vi "sub vi - Read Analog All v9.4.vi"() -> (0 "DATA0":dbl[](graph), 2 "Analog loop time":dbl, 3 "array GRAPH":dynamicdata[](array[waveform]), 4 "LAB01":T2, 5 "DATA1":dbl[](graph), 6 "LAB02":T3, 7 "DATA2":dbl[](graph), 8 "LAB03":T4, 10 "LAB04":T5, 13 "deg C":dbl, 14 "USB Error":bool[](array[boolean]), 15 "LAB05":T6)   [LabVIEW 2013]
uses:
  <vilib>/addons/Electrical Power/Basic/NI_EP_Basic.lvlib
  <vilib>/addons/Electrical Power/Basic/Measurement/Power (1 Channel).vi
  <vilib>/addons/Electrical Power/Basic/Measurement/RMS (N Channels).vi
  <vilib>/measure/NI_MAPro.lvlib
  <vilib>/measure/mascope.llb/Amplitude and Levels 1 chan.vi
  program files/Global display 3.vi
  <vilib>/addons/Electrical Power/Basic/Measurement/RMS (1 Channel).vi
panel:
  in  "Tab Control":T1(tab)
  out "LAB01-2 (PF)":dbl
  out "LAB01-1 (PF)":dbl
  out "LAB01-2 (V)":dbl
  out "LAB01-2 (A)":dbl
  out "LAB01-1 (V)":dbl
  out "LAB01-1 (A)":dbl
  out "LAB01-2 (GRAPH)":dynamicdata(graph)
  out "LAB01-1 (GRAPH)":dynamicdata(graph)
  out "LAB02-2 (PF)":dbl
  out "LAB02-1 (PF)":dbl
  out "LAB02-2 (V)":dbl
  out "LAB02-2 (A)":dbl
  out "LAB02-1 (V)":dbl
  out "LAB02-1 (A)":dbl
  out "LAB02-2 (GRAPH)":dynamicdata(graph)
  out "LAB02-1 (GRAPH)":dynamicdata(graph)
  out "LAB03-2 (PF)":dbl
  out "LAB03-1 (PF)":dbl
  out "LAB03-2 (V)":dbl
  out "LAB03-2 (A)":dbl
  out "LAB03-1 (V)":dbl
  out "LAB03-1 (A)":dbl
  out "LAB03-2 (GRAPH)":dynamicdata(graph)
  out "LAB03-1 (GRAPH)":dynamicdata(graph)
  out "LAB04-2 (PF)":dbl
  out "LAB04-1 (PF)":dbl
  out "LAB04-2 (V)":dbl
  out "LAB04-2 (A)":dbl
  out "LAB04-1 (V)":dbl
  out "LAB04-1 (A)":dbl
  out "LAB04-1 (GRAPH)":dynamicdata(graph)
  out "LAB04-2 (GRAPH)":dynamicdata(graph)
  out "LAB05-2 (PF)":dbl
  out "LAB05-1 (PF)":dbl
  out "LAB05-2 (V)":dbl
  out "LAB05-2 (A)":dbl
  out "LAB05-1 (V)":dbl
  out "LAB05-1 (A)":dbl
  out "LAB05-1 (GRAPH)":dynamicdata(graph)
  out "LAB05-2 (GRAPH)":dynamicdata(graph)
  out "A1 error":errorcluster
  out "array ERROR":errorcluster[](array[cluster])
  out "AI2-OFF":waveform(dbl)[](graph)
  out "AI2-ON":waveform(dbl)[](graph)
  out "AI1-OFF":waveform(dbl)[](graph)
  out "AI1-ON":waveform(dbl)[](graph)
  out "AI0-OFF":waveform(dbl)[](graph)
  out "AI0-ON":waveform(dbl)[](graph)
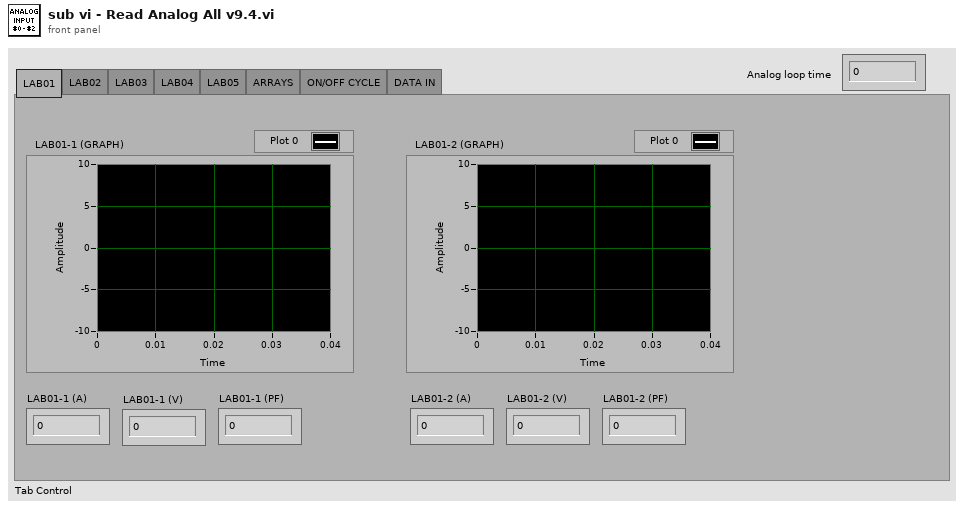
[diagram p1: front panel]
types:
  T1 = enum32{"LAB01", "LAB02", "LAB03", "LAB04", "LAB05", "ARRAYS", "ON/OFF CYCLE", "DATA IN"}
  T2 = cluster{"LAB01-1 (A)":dbl, "LAB01-1 (V)":dbl, "LAB01-1 (PF)":dbl, "LAB01-2 (A)":dbl, "LAB01-2 (V)":dbl, "LAB01-2 (PF)":dbl}
  T3 = cluster{"LAB02-1 (A)":dbl, "LAB02-1 (V)":dbl, "LAB02-1 (PF)":dbl, "LAB02-2 (A)":dbl, "LAB02-2 (V)":dbl, "LAB02-2 (PF)":dbl}
  T4 = cluster{"LAB03-1 (A)":dbl, "LAB03-1 (V)":dbl, "LAB03-1 (PF)":dbl, "LAB03-2 (A)":dbl, "LAB03-2 (V)":dbl, "LAB03-2 (PF)":dbl}
  T5 = cluster{"LAB04-1 (A)":dbl, "LAB04-1 (V)":dbl, "LAB04-1 (PF)":dbl, "LAB04-2 (A)":dbl, "LAB04-2 (V)":dbl, "LAB04-2 (PF)":dbl}
  T6 = cluster{"LAB05-1 (A)":dbl, "LAB05-1 (V)":dbl, "LAB05-1 (PF)":dbl, "LAB05-2 (A)":dbl, "LAB05-2 (V)":dbl, "LAB05-2 (PF)":dbl}
  T7 = typedef "NI_EP_Basic.lvlib/basic_Power Value.ctl" = cluster{"active power [W]":dbl, "apparent power [VA]":dbl, "reactive power [VAR]":dbl, "power factor":dbl}
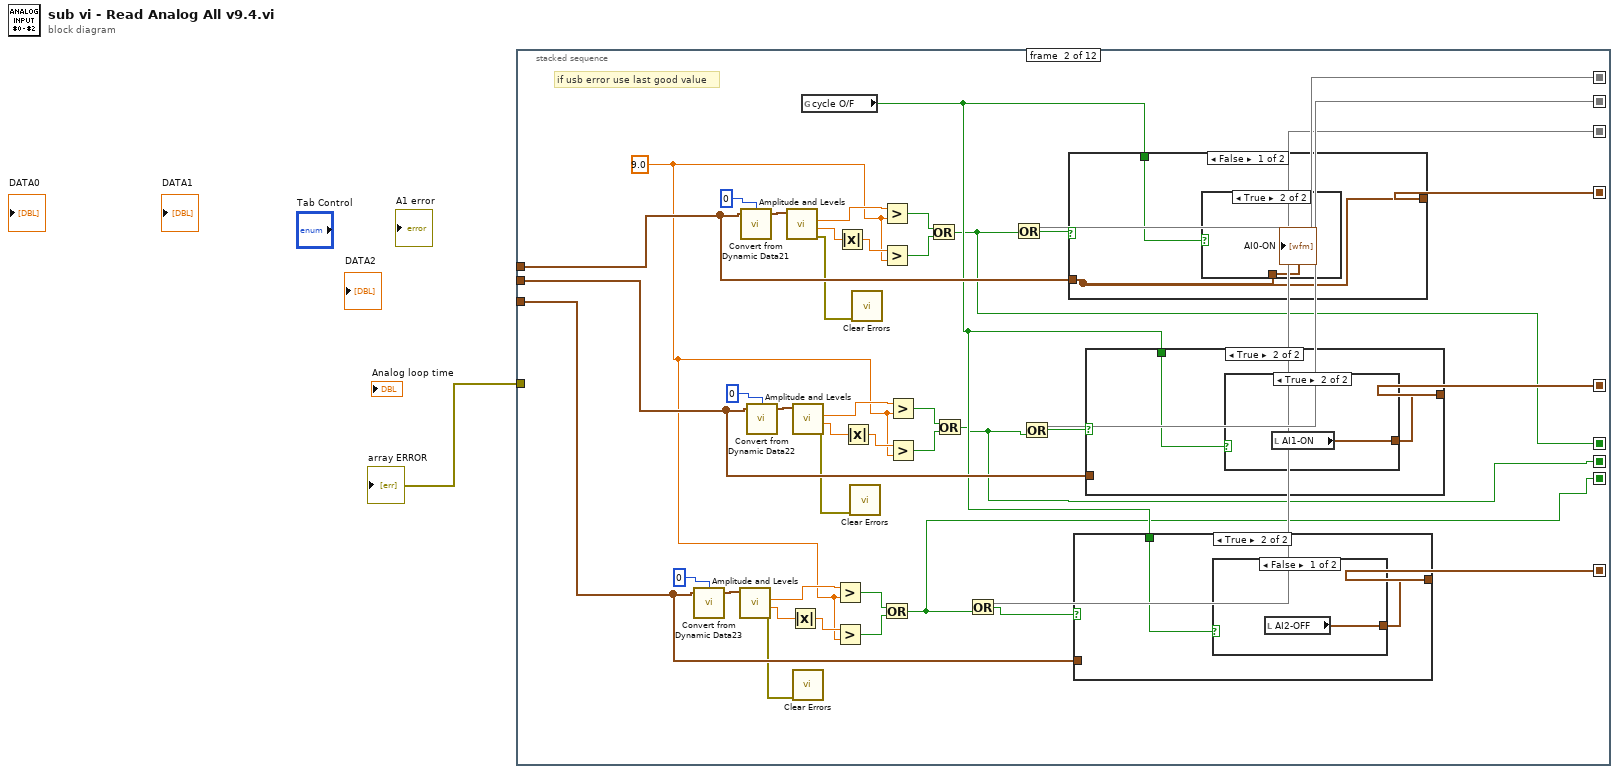
[diagram p0: block diagram]
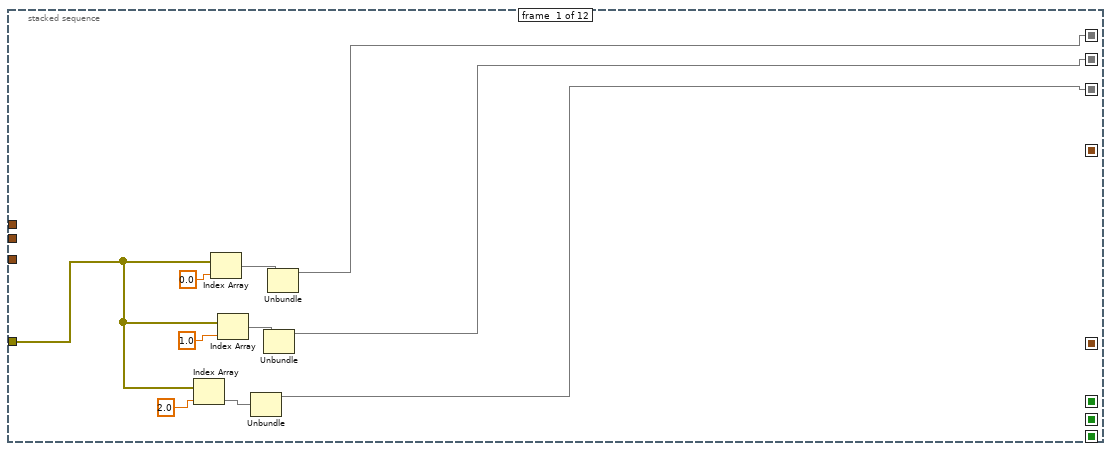
[diagram p2: hidden frame]
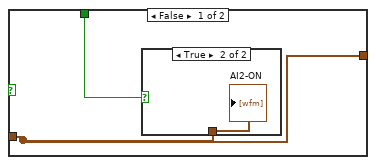
[diagram p3: hidden frame]
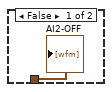
[diagram p4: hidden frame]
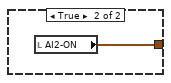
[diagram p5: hidden frame]
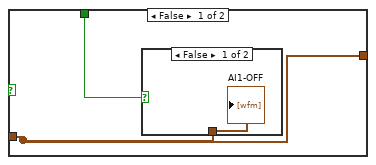
[diagram p6: hidden frame]
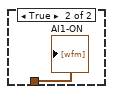
[diagram p7: hidden frame]
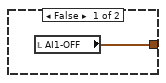
[diagram p8: hidden frame]
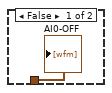
[diagram p9: hidden frame]
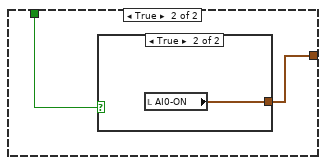
[diagram p10: hidden frame]
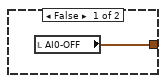
[diagram p11: hidden frame]
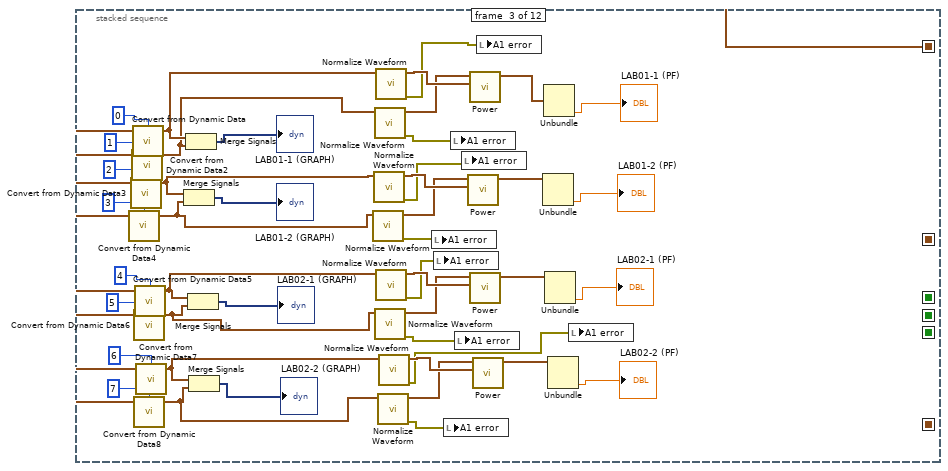
[diagram p12: hidden frame]
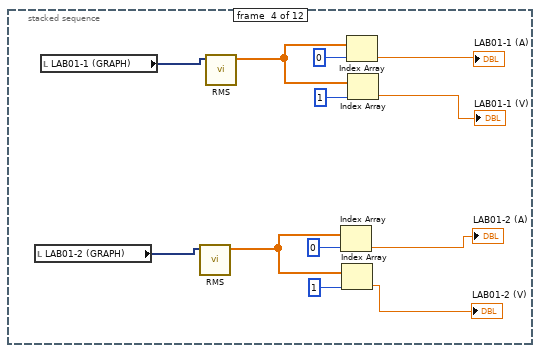
[diagram p13: hidden frame]
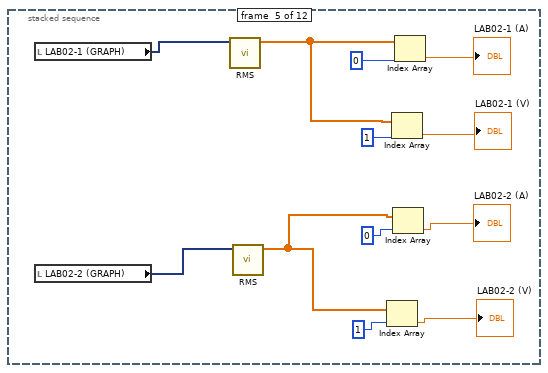
[diagram p14: hidden frame]
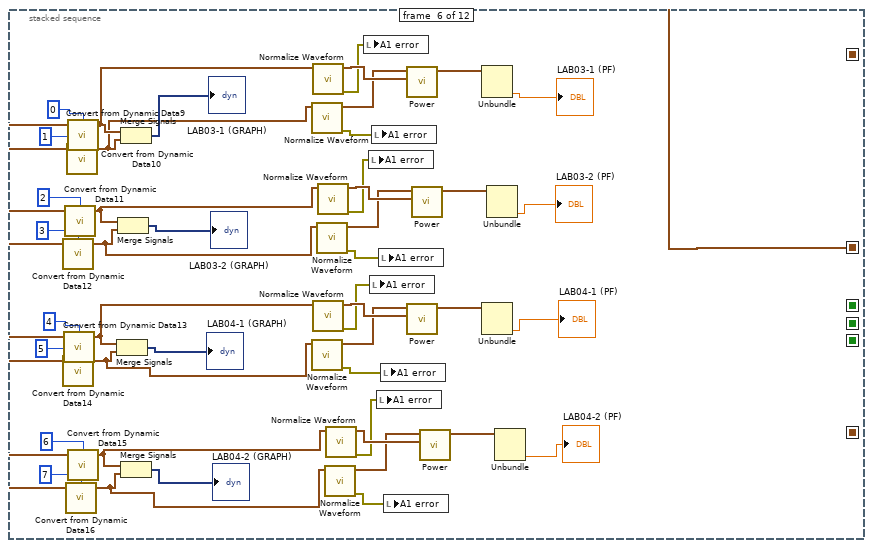
[diagram p15: hidden frame]
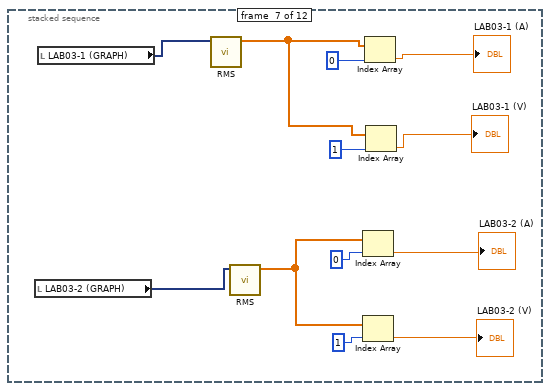
[diagram p16: hidden frame]
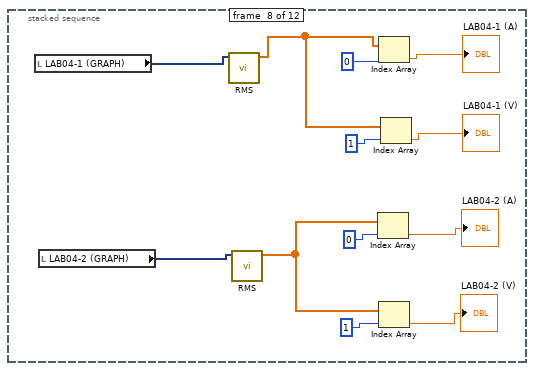
[diagram p17: hidden frame]
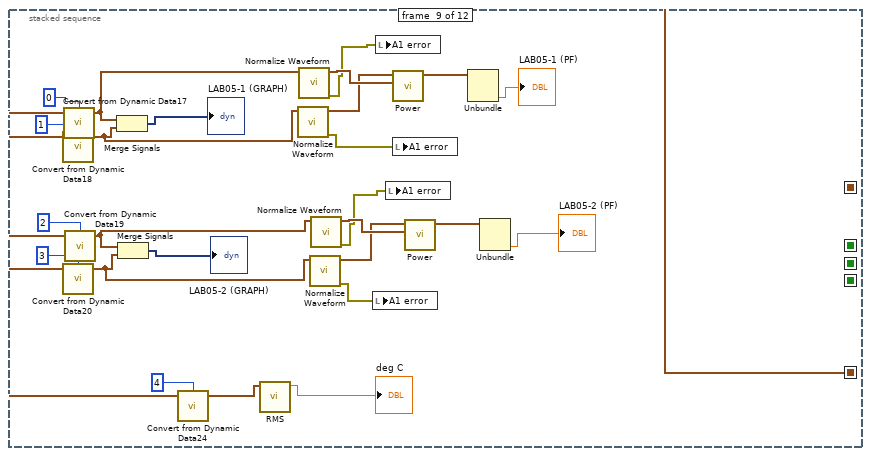
[diagram p18: hidden frame]
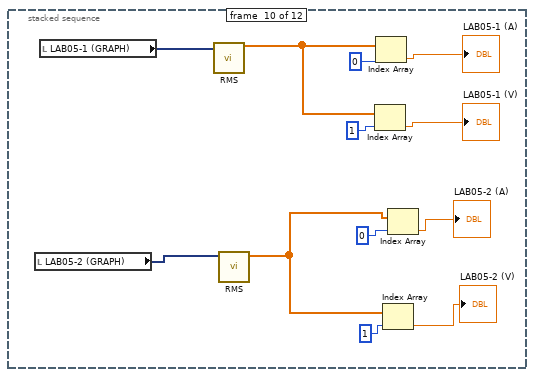
[diagram p19: hidden frame]
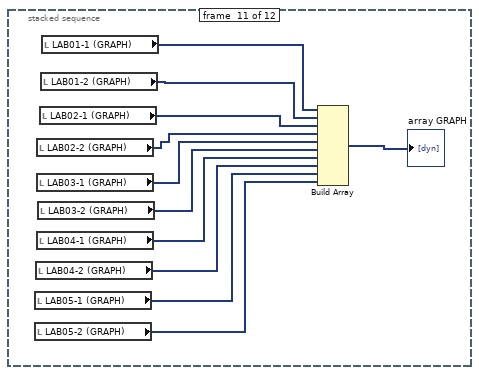
[diagram p20: hidden frame]
diagram:
  n1 = stacked-sequence {
    seq-local: [w13 _ _ _ _ _ _ _ _ _ _ _] -> [_ w23 _ _ _ _ _ _ _ _ _ w273]
    seq-local: [w10 _ _ _ _ _ _ _ _ _ _ _] -> [_ w22 _ _ _ _ _ _ _ _ _ w272]
    seq-local: [w6 _ _ _ _ _ _ _ _ _ _ _] -> [_ w19 _ _ _ _ _ _ _ _ _ w271]
    seq-local: [_ w49 _ _ _ _ _ _ _ _ _ _] -> [_ _ w125 _ _ _ _ _ _ _ _ _]
    seq-local: [_ w39 _ _ _ _ _ _ _ _ _ _] -> [_ _ _ _ _ w194 _ _ _ _ _ _]
    seq-local: [_ w28 _ _ _ _ _ _ _ _ _ _] -> [_ _ _ _ _ _ _ _ w244 _ _ _]
    seq-local: [_ w18 _ _ _ _ _ _ _ _ _ _] -> [_ _ _ _ _ _ _ _ _ _ _ w270]
    seq-local: [_ w17 _ _ _ _ _ _ _ _ _ _] -> [_ _ _ _ _ _ _ _ _ _ _ w269]
    seq-local: [_ w16 _ _ _ _ _ _ _ _ _ _] -> [_ _ _ _ _ _ _ _ _ _ _ w268]
    tunnel: [_ w48 _ _ _ _ _ _ _ _ _ _] -> w5
    tunnel: [_ w40 _ _ _ _ _ _ _ _ _ _] -> w4
    tunnel: [_ w31 _ _ _ _ _ _ _ _ _ _] -> w3
    tunnel: [w7 _ _ _ _ _ _ _ _ _ _ _] -> w1
    frame #0 {
      n2 = Index Array(array=w7, index=2.0) -> (element=w8)
      n3 = Index Array(array=w7, index=0.0) -> (element=w14)
      n4 = Index Array(array=w7, index=1.0) -> (element=w11)
      n5 = Unbundle(w8) -> (w6)  [unwired: 2 out]
      n6 = Unbundle(w11) -> (w10)  [unwired: 2 out]
      n7 = Unbundle(w14) -> (w13)  [unwired: 2 out]
    }
    frame #1 {
      w30 = 9.0
      # "if usb error use last good value"
      n8 = call "Convert from Dynamic Data23"("Dynamic Data Type"=w31, "Channel"=0) -> ("Waveform"=w37:waveform(dbl))  [unwired: 2 in]
      n9 = call-poly <vilib>:"Amplitude and Levels.vi"("signal in"=w37) -> ("error out"=w25:errorcluster, "low state level"=w36:dbl, "high state level"=w35:dbl)  [unwired: 7 in, 1 out]
      n10 = call "Convert from Dynamic Data21"("Dynamic Data Type"=w48, "Channel"=0) -> ("Waveform"=w55:waveform(dbl))  [unwired: 2 in]
      n11 = call "Convert from Dynamic Data22"("Dynamic Data Type"=w40, "Channel"=0) -> ("Waveform"=w46:waveform(dbl))  [unwired: 2 in]
      n12 = call-poly <vilib>:"Amplitude and Levels.vi"("signal in"=w55) -> ("error out"=w27:errorcluster, "low state level"=w54:dbl, "high state level"=w53:dbl)  [unwired: 7 in, 1 out]
      n13 = Absolute Value(x=w36) -> (abs(x)=w34:dbl)
      n14 = call-poly <vilib>:"Amplitude and Levels.vi"("signal in"=w46) -> ("error out"=w26:errorcluster, "low state level"=w45:dbl, "high state level"=w44:dbl)  [unwired: 7 in, 1 out]
      n15 = call <vilib>:"Clear Errors.vi"("error in (no error)"=w25) -> ()  [unwired: 6 in, 1 out]
      n16 = global read "Global display 3.vi" "cycle O/F"() -> (w29:bool)
      n17 = Greater?(x=w35, y=w30) -> (0:w33:bool)
      n18 = Greater?(x=w34, y=w30) -> (0:w32:bool)
      n19 = Absolute Value(x=w54) -> (abs(x)=w52:dbl)
      n20 = Absolute Value(x=w45) -> (abs(x)=w43:dbl)
      n21 = call <vilib>:"Clear Errors.vi"("error in (no error)"=w26) -> ()  [unwired: 6 in, 1 out]
      n22 = call <vilib>:"Clear Errors.vi"("error in (no error)"=w27) -> ()  [unwired: 6 in, 1 out]
      n23 = Greater?(x=w53, y=w30) -> (0:w51:bool)
      n24 = Greater?(x=w52, y=w30) -> (0:w50:bool)
      n25 = Or(x=w33, y=w32) -> (x .or. y?=w16:bool)
      n26 = Greater?(x=w44, y=w30) -> (0:w42:bool)
      n27 = Greater?(x=w43, y=w30) -> (0:w41:bool)
      n28 = Or(x=w51, y=w50) -> (x .or. y?=w18:bool)
      n29 = Or(x=w42, y=w41) -> (x .or. y?=w17:bool)
      n30 = Or(x=w19, y=w16) -> (x .or. y?=w20:bool)
      n31 = Or(x=w23, y=w18) -> (x .or. y?=w24:bool)
      n32 = Or(x=w22, y=w17) -> (x .or. y?=w21:bool)
      n33 = case shown="False" w24 {
        tunnel: w29 -> [w74 w78]
        tunnel: [w73 w77] -> w49
        tunnel: w48 -> [w73 _]
        frame False {
          n34 = case shown="True" w74 {
            tunnel: w73 -> [w75 w76]
            frame False {
              "AI0-OFF" <- w75
            }
            frame True {
              "AI0-ON" <- w76
            }
          }
        }
        frame True {
          n35 = case shown="True" w78 {
            tunnel: [w79 w80] -> w77
            frame False {
              n36 = local read "AI0-OFF"() -> (w79:waveform(dbl)[])
            }
            frame True {
              n37 = local read "AI0-ON"() -> (w80:waveform(dbl)[])
            }
          }
        }
      }
      n38 = case shown="True" w20 {
        tunnel: w29 -> [w58 w62]
        tunnel: [w57 w61] -> w28
        tunnel: w31 -> [w57 _]
        frame False {
          n39 = case shown="True" w58 {
            tunnel: w57 -> [w59 w60]
            frame False {
              "AI2-OFF" <- w59
            }
            frame True {
              "AI2-ON" <- w60
            }
          }
        }
        frame True {
          n40 = case shown="False" w62 {
            tunnel: [w63 w64] -> w61
            frame False {
              n41 = local read "AI2-OFF"() -> (w63:waveform(dbl)[])
            }
            frame True {
              n42 = local read "AI2-ON"() -> (w64:waveform(dbl)[])
            }
          }
        }
      }
      n43 = case shown="True" w21 {
        tunnel: w29 -> [w66 w70]
        tunnel: [w65 w69] -> w39
        tunnel: w40 -> [w65 _]
        frame False {
          n44 = case shown="False" w66 {
            tunnel: w65 -> [w67 w68]
            frame False {
              "AI1-OFF" <- w67
            }
            frame True {
              "AI1-ON" <- w68
            }
          }
        }
        frame True {
          n45 = case shown="True" w70 {
            tunnel: [w71 w72] -> w69
            frame False {
              n46 = local read "AI1-OFF"() -> (w71:waveform(dbl)[])
            }
            frame True {
              n47 = local read "AI1-ON"() -> (w72:waveform(dbl)[])
            }
          }
        }
      }
    }
    frame #2 {
      n48 = call "Convert from Dynamic Data4"("Dynamic Data Type"=w125, "Channel"=3) -> ("Waveform"=w101:waveform(dbl))  [unwired: 2 in]
      n49 = call "Convert from Dynamic Data3"("Dynamic Data Type"=w125, "Channel"=2) -> ("Waveform"=w102:waveform(dbl))  [unwired: 2 in]
      n50 = call "Convert from Dynamic Data2"("Dynamic Data Type"=w125, "Channel"=1) -> ("Waveform"=w111:waveform(dbl))  [unwired: 2 in]
      n51 = call "Convert from Dynamic Data"("Dynamic Data Type"=w125, "Channel"=0) -> ("Waveform"=w112:waveform(dbl))  [unwired: 2 in]
      n52 = call "Convert from Dynamic Data6"("Dynamic Data Type"=w125, "Channel"=5) -> ("Waveform"=w96:waveform(dbl))  [unwired: 2 in]
      n53 = call "Convert from Dynamic Data8"("Dynamic Data Type"=w125, "Channel"=7) -> ("Waveform"=w90:waveform(dbl))  [unwired: 2 in]
      n54 = call "Convert from Dynamic Data5"("Dynamic Data Type"=w125, "Channel"=4) -> ("Waveform"=w97:waveform(dbl))  [unwired: 2 in]
      n55 = call "Convert from Dynamic Data7"("Dynamic Data Type"=w125, "Channel"=6) -> ("Waveform"=w91:waveform(dbl))  [unwired: 2 in]
      n56 = Merge Signals(w102, w101) -> (→"LAB01-2 (GRAPH)":dynamicdata)
      n57 = Merge Signals(w112, w111) -> (→"LAB01-1 (GRAPH)":dynamicdata)
      n58 = Merge Signals(w97, w96) -> (→"LAB02-1 (GRAPH)":dynamicdata)
      n59 = Merge Signals(w91, w90) -> (→"LAB02-2 (GRAPH)":dynamicdata)
      n60 = call <vilib>:"Normalize Waveform.vi"("waveform in"=w101) -> ("error out"=w85:errorcluster, "normalized waveform"=w105:waveform(dbl))  [unwired: 7 in, 2 out]
      n61 = call <vilib>:"Normalize Waveform.vi"("waveform in"=w102) -> ("error out"=w86:errorcluster, "normalized waveform"=w106:waveform(dbl))  [unwired: 7 in, 2 out]
      n62 = call <vilib>:"Normalize Waveform.vi"("waveform in"=w111) -> ("error out"=w87:errorcluster, "normalized waveform"=w109:waveform(dbl))  [unwired: 7 in, 2 out]
      n63 = call <vilib>:"Normalize Waveform.vi"("waveform in"=w96) -> ("error out"=w83:errorcluster, "normalized waveform"=w99:waveform(dbl))  [unwired: 7 in, 2 out]
      n64 = call <vilib>:"Normalize Waveform.vi"("waveform in"=w112) -> ("error out"=w88:errorcluster, "normalized waveform"=w110:waveform(dbl))  [unwired: 7 in, 2 out]
      n65 = call <vilib>:"Normalize Waveform.vi"("waveform in"=w97) -> ("error out"=w84:errorcluster, "normalized waveform"=w100:waveform(dbl))  [unwired: 7 in, 2 out]
      n66 = call <vilib>:"Normalize Waveform.vi"("waveform in"=w90) -> ("error out"=w81:errorcluster, "normalized waveform"=w93:waveform(dbl))  [unwired: 7 in, 2 out]
      n67 = call <vilib>:"Normalize Waveform.vi"("waveform in"=w91) -> ("error out"=w82:errorcluster, "normalized waveform"=w94:waveform(dbl))  [unwired: 7 in, 2 out]
      n68 = local write "A1 error"(w85) -> ()
      n69 = local write "A1 error"(w84) -> ()
      n70 = local write "A1 error"(w81) -> ()
      n71 = local write "A1 error"(w87) -> ()
      n72 = local write "A1 error"(w83) -> ()
      n73 = local write "A1 error"(w86) -> ()
      n74 = call-poly <vilib>:"Power.vi"("current waveform"=w106, "voltage waveform"=w105) -> ("power value"=w104:T7)  [unwired: 8 in, 1 out]
      n75 = call-poly <vilib>:"Power.vi"("current waveform"=w110, "voltage waveform"=w109) -> ("power value"=w108:T7)  [unwired: 8 in, 1 out]
      n76 = call-poly <vilib>:"Power.vi"("current waveform"=w100, "voltage waveform"=w99) -> ("power value"=w98:T7)  [unwired: 8 in, 1 out]
      n77 = call-poly <vilib>:"Power.vi"("current waveform"=w94, "voltage waveform"=w93) -> ("power value"=w92:T7)  [unwired: 8 in, 1 out]
      n78 = local write "A1 error"(w88) -> ()
      n79 = Unbundle(w104) -> ("power factor"=→"LAB01-2 (PF)":dbl)  [unwired: 3 out]
      n80 = Unbundle(w108) -> ("power factor"=→"LAB01-1 (PF)":dbl)  [unwired: 3 out]
      n81 = Unbundle(w98) -> ("power factor"=→"LAB02-1 (PF)":dbl)  [unwired: 3 out]
      n82 = Unbundle(w92) -> ("power factor"=→"LAB02-2 (PF)":dbl)  [unwired: 3 out]
      n83 = local write "A1 error"(w82) -> ()
    }
    frame #3 {
      n84 = local read "LAB01-2 (GRAPH)"() -> (w134:dynamicdata)
      n85 = local read "LAB01-1 (GRAPH)"() -> (w128:dynamicdata)
      n86 = call-poly <vilib>:"RMS.vi"("waveforms"=w134) -> ("RMS values"=w133:dbl[])  [unwired: 9 in, 1 out]
      n87 = call-poly <vilib>:"RMS.vi"("waveforms"=w128) -> ("RMS values"=w137:dbl[])  [unwired: 9 in, 1 out]
      n88 = Index Array(array=w133, index=0) -> (element=→"LAB01-2 (A)":dbl)
      n89 = Index Array(array=w133, index=1) -> (element=→"LAB01-2 (V)":dbl)
      n90 = Index Array(array=w137, index=0) -> (element=→"LAB01-1 (A)":dbl)
      n91 = Index Array(array=w137, index=1) -> (element=→"LAB01-1 (V)":dbl)
    }
    frame #4 {
      n92 = local read "LAB02-1 (GRAPH)"() -> (w145:dynamicdata)
      n93 = local read "LAB02-2 (GRAPH)"() -> (w141:dynamicdata)
      n94 = call-poly <vilib>:"RMS.vi"("waveforms"=w145) -> ("RMS values"=w144:dbl[])  [unwired: 9 in, 1 out]
      n95 = call-poly <vilib>:"RMS.vi"("waveforms"=w141) -> ("RMS values"=w140:dbl[])  [unwired: 9 in, 1 out]
      n96 = Index Array(array=w140, index=1) -> (element=→"LAB02-2 (V)":dbl)
      n97 = Index Array(array=w144, index=1) -> (element=→"LAB02-1 (V)":dbl)
      n98 = Index Array(array=w140, index=0) -> (element=→"LAB02-2 (A)":dbl)
      n99 = Index Array(array=w144, index=0) -> (element=→"LAB02-1 (A)":dbl)
    }
    frame #5 {
      n100 = call "Convert from Dynamic Data12"("Dynamic Data Type"=w194, "Channel"=3) -> ("Waveform"=w171:waveform(dbl))  [unwired: 2 in]
      n101 = call "Convert from Dynamic Data14"("Dynamic Data Type"=w194, "Channel"=5) -> ("Waveform"=w165:waveform(dbl))  [unwired: 2 in]
      n102 = call "Convert from Dynamic Data13"("Dynamic Data Type"=w194, "Channel"=4) -> ("Waveform"=w166:waveform(dbl))  [unwired: 2 in]
      n103 = call "Convert from Dynamic Data11"("Dynamic Data Type"=w194, "Channel"=2) -> ("Waveform"=w172:waveform(dbl))  [unwired: 2 in]
      n104 = call "Convert from Dynamic Data16"("Dynamic Data Type"=w194, "Channel"=7) -> ("Waveform"=w159:waveform(dbl))  [unwired: 2 in]
      n105 = call "Convert from Dynamic Data10"("Dynamic Data Type"=w194, "Channel"=1) -> ("Waveform"=w177:waveform(dbl))  [unwired: 2 in]
      n106 = call "Convert from Dynamic Data9"("Dynamic Data Type"=w194, "Channel"=0) -> ("Waveform"=w178:waveform(dbl))  [unwired: 2 in]
      n107 = call "Convert from Dynamic Data15"("Dynamic Data Type"=w194, "Channel"=6) -> ("Waveform"=w160:waveform(dbl))  [unwired: 2 in]
      n108 = Merge Signals(w166, w165) -> (→"LAB04-1 (GRAPH)":dynamicdata)
      n109 = Merge Signals(w172, w171) -> (→"LAB03-2 (GRAPH)":dynamicdata)
      n110 = Merge Signals(w178, w177) -> (→"LAB03-1 (GRAPH)":dynamicdata)
      n111 = Merge Signals(w160, w159) -> (→"LAB04-2 (GRAPH)":dynamicdata)
      n112 = call <vilib>:"Normalize Waveform.vi"("waveform in"=w177) -> ("error out"=w156:errorcluster, "normalized waveform"=w180:waveform(dbl))  [unwired: 7 in, 2 out]
      n113 = call <vilib>:"Normalize Waveform.vi"("waveform in"=w165) -> ("error out"=w152:errorcluster, "normalized waveform"=w168:waveform(dbl))  [unwired: 7 in, 2 out]
      n114 = call <vilib>:"Normalize Waveform.vi"("waveform in"=w178) -> ("error out"=w157:errorcluster, "normalized waveform"=w181:waveform(dbl))  [unwired: 7 in, 2 out]
      n115 = call <vilib>:"Normalize Waveform.vi"("waveform in"=w166) -> ("error out"=w153:errorcluster, "normalized waveform"=w169:waveform(dbl))  [unwired: 7 in, 2 out]
      n116 = call <vilib>:"Normalize Waveform.vi"("waveform in"=w171) -> ("error out"=w154:errorcluster, "normalized waveform"=w174:waveform(dbl))  [unwired: 7 in, 2 out]
      n117 = call <vilib>:"Normalize Waveform.vi"("waveform in"=w172) -> ("error out"=w155:errorcluster, "normalized waveform"=w175:waveform(dbl))  [unwired: 7 in, 2 out]
      n118 = call <vilib>:"Normalize Waveform.vi"("waveform in"=w159) -> ("error out"=w150:errorcluster, "normalized waveform"=w162:waveform(dbl))  [unwired: 7 in, 2 out]
      n119 = call <vilib>:"Normalize Waveform.vi"("waveform in"=w160) -> ("error out"=w151:errorcluster, "normalized waveform"=w163:waveform(dbl))  [unwired: 7 in, 2 out]
      n120 = local write "A1 error"(w157) -> ()
      n121 = local write "A1 error"(w155) -> ()
      n122 = local write "A1 error"(w153) -> ()
      n123 = local write "A1 error"(w156) -> ()
      n124 = local write "A1 error"(w151) -> ()
      n125 = local write "A1 error"(w154) -> ()
      n126 = local write "A1 error"(w152) -> ()
      n127 = local write "A1 error"(w150) -> ()
      n128 = call-poly <vilib>:"Power.vi"("current waveform"=w181, "voltage waveform"=w180) -> ("power value"=w179:T7)  [unwired: 8 in, 1 out]
      n129 = call-poly <vilib>:"Power.vi"("current waveform"=w169, "voltage waveform"=w168) -> ("power value"=w167:T7)  [unwired: 8 in, 1 out]
      n130 = call-poly <vilib>:"Power.vi"("current waveform"=w175, "voltage waveform"=w174) -> ("power value"=w173:T7)  [unwired: 8 in, 1 out]
      n131 = call-poly <vilib>:"Power.vi"("current waveform"=w163, "voltage waveform"=w162) -> ("power value"=w161:T7)  [unwired: 8 in, 1 out]
      n132 = Unbundle(w179) -> ("power factor"=→"LAB03-1 (PF)":dbl)  [unwired: 3 out]
      n133 = Unbundle(w167) -> ("power factor"=→"LAB04-1 (PF)":dbl)  [unwired: 3 out]
      n134 = Unbundle(w173) -> ("power factor"=→"LAB03-2 (PF)":dbl)  [unwired: 3 out]
      n135 = Unbundle(w161) -> ("power factor"=→"LAB04-2 (PF)":dbl)  [unwired: 3 out]
    }
    frame #6 {
      n136 = local read "LAB03-2 (GRAPH)"() -> (w201:dynamicdata)
      n137 = local read "LAB03-1 (GRAPH)"() -> (w202:dynamicdata)
      n138 = call-poly <vilib>:"RMS.vi"("waveforms"=w202) -> ("RMS values"=w200:dbl[])  [unwired: 9 in, 1 out]
      n139 = call-poly <vilib>:"RMS.vi"("waveforms"=w201) -> ("RMS values"=w197:dbl[])  [unwired: 9 in, 1 out]
      n140 = Index Array(array=w197, index=0) -> (element=→"LAB03-2 (A)":dbl)
      n141 = Index Array(array=w197, index=1) -> (element=→"LAB03-2 (V)":dbl)
      n142 = Index Array(array=w200, index=0) -> (element=→"LAB03-1 (A)":dbl)
      n143 = Index Array(array=w200, index=1) -> (element=→"LAB03-1 (V)":dbl)
    }
    frame #7 {
      n144 = local read "LAB04-1 (GRAPH)"() -> (w214:dynamicdata)
      n145 = local read "LAB04-2 (GRAPH)"() -> (w210:dynamicdata)
      n146 = call-poly <vilib>:"RMS.vi"("waveforms"=w214) -> ("RMS values"=w213:dbl[])  [unwired: 9 in, 1 out]
      n147 = call-poly <vilib>:"RMS.vi"("waveforms"=w210) -> ("RMS values"=w209:dbl[])  [unwired: 9 in, 1 out]
      n148 = Index Array(array=w209, index=0) -> (element=→"LAB04-2 (A)":dbl)
      n149 = Index Array(array=w213, index=0) -> (element=→"LAB04-1 (A)":dbl)
      n150 = Index Array(array=w209, index=1) -> (element=→"LAB04-2 (V)":dbl)
      n151 = Index Array(array=w213, index=1) -> (element=→"LAB04-1 (V)":dbl)
    }
    frame #8 {
      n152 = call "Convert from Dynamic Data18"("Dynamic Data Type"=w244, "Channel"=1) -> ("Waveform"=w233:waveform(dbl))  [unwired: 2 in]
      n153 = call "Convert from Dynamic Data20"("Dynamic Data Type"=w244, "Channel"=3) -> ("Waveform"=w227:waveform(dbl))  [unwired: 2 in]
      n154 = call "Convert from Dynamic Data17"("Dynamic Data Type"=w244, "Channel"=0) -> ("Waveform"=w234:waveform(dbl))  [unwired: 2 in]
      n155 = call "Convert from Dynamic Data19"("Dynamic Data Type"=w244, "Channel"=2) -> ("Waveform"=w228:waveform(dbl))  [unwired: 2 in]
      n156 = Merge Signals(w234, w233) -> (→"LAB05-1 (GRAPH)":dynamicdata)
      n157 = Merge Signals(w228, w227) -> (→"LAB05-2 (GRAPH)":dynamicdata)
      n158 = call "Convert from Dynamic Data24"("Dynamic Data Type"=w244, "Channel"=4) -> ("Waveform"=w220:waveform(dbl))  [unwired: 2 in]
      n159 = call-poly <vilib>:"RMS.vi"("waveform"=w220) -> ("RMS value"=→"deg C":dbl)  [unwired: 9 in, 1 out]
      n160 = call <vilib>:"Normalize Waveform.vi"("waveform in"=w233) -> ("error out"=w225:errorcluster, "normalized waveform"=w236:waveform(dbl))  [unwired: 7 in, 2 out]
      n161 = call <vilib>:"Normalize Waveform.vi"("waveform in"=w234) -> ("error out"=w224:errorcluster, "normalized waveform"=w237:waveform(dbl))  [unwired: 7 in, 2 out]
      n162 = call <vilib>:"Normalize Waveform.vi"("waveform in"=w227) -> ("error out"=w223:errorcluster, "normalized waveform"=w230:waveform(dbl))  [unwired: 7 in, 2 out]
      n163 = call <vilib>:"Normalize Waveform.vi"("waveform in"=w228) -> ("error out"=w222:errorcluster, "normalized waveform"=w231:waveform(dbl))  [unwired: 7 in, 2 out]
      n164 = local write "A1 error"(w223) -> ()
      n165 = local write "A1 error"(w224) -> ()
      n166 = local write "A1 error"(w222) -> ()
      n167 = call-poly <vilib>:"Power.vi"("current waveform"=w237, "voltage waveform"=w236) -> ("power value"=w235:T7)  [unwired: 8 in, 1 out]
      n168 = local write "A1 error"(w225) -> ()
      n169 = call-poly <vilib>:"Power.vi"("current waveform"=w231, "voltage waveform"=w230) -> ("power value"=w229:T7)  [unwired: 8 in, 1 out]
      n170 = Unbundle(w235) -> ("power factor"=→"LAB05-1 (PF)":dbl)  [unwired: 3 out]
      n171 = Unbundle(w229) -> ("power factor"=→"LAB05-2 (PF)":dbl)  [unwired: 3 out]
    }
    frame #9 {
      n172 = local read "LAB05-2 (GRAPH)"() -> (w251:dynamicdata)
      n173 = local read "LAB05-1 (GRAPH)"() -> (w252:dynamicdata)
      n174 = call-poly <vilib>:"RMS.vi"("waveforms"=w252) -> ("RMS values"=w250:dbl[])  [unwired: 9 in, 1 out]
      n175 = call-poly <vilib>:"RMS.vi"("waveforms"=w251) -> ("RMS values"=w249:dbl[])  [unwired: 9 in, 1 out]
      n176 = Index Array(array=w250, index=1) -> (element=→"LAB05-1 (V)":dbl)
      n177 = Index Array(array=w250, index=0) -> (element=→"LAB05-1 (A)":dbl)
      n178 = Index Array(array=w249, index=1) -> (element=→"LAB05-2 (V)":dbl)
      n179 = Index Array(array=w249, index=0) -> (element=→"LAB05-2 (A)":dbl)
    }
    frame #10 {
      n180 = local read "LAB05-1 (GRAPH)"() -> (w259:dynamicdata)
      n181 = local read "LAB05-2 (GRAPH)"() -> (w258:dynamicdata)
      n182 = local read "LAB04-2 (GRAPH)"() -> (w260:dynamicdata)
      n183 = local read "LAB02-2 (GRAPH)"() -> (w264:dynamicdata)
      n184 = local read "LAB03-1 (GRAPH)"() -> (w263:dynamicdata)
      n185 = local read "LAB04-1 (GRAPH)"() -> (w261:dynamicdata)
      n186 = local read "LAB03-2 (GRAPH)"() -> (w262:dynamicdata)
      n187 = local read "LAB02-1 (GRAPH)"() -> (w265:dynamicdata)
      n188 = local read "LAB01-2 (GRAPH)"() -> (w266:dynamicdata)
      n189 = local read "LAB01-1 (GRAPH)"() -> (w267:dynamicdata)
      n190 = Build Array(w267, w266, w265, w264, w263, w262, w261, w260, w259, w258) -> (→"array GRAPH":dynamicdata[])
    }
    frame #11 {
      n191 = local read "LAB03-2 (PF)"() -> (w292:dbl)
      n192 = local read "LAB03-1 (PF)"() -> (w295:dbl)
      n193 = local read "LAB03-1 (A)"() -> (w297:dbl)
      n194 = local read "LAB03-1 (V)"() -> (w296:dbl)
      n195 = local read "LAB03-2 (A)"() -> (w294:dbl)
      n196 = local read "LAB03-2 (V)"() -> (w293:dbl)
      n197 = local read "LAB01-1 (PF)"() -> (w302:dbl)
      n198 = local read "LAB01-2 (PF)"() -> (w299:dbl)
      n199 = local read "LAB01-1 (V)"() -> (w303:dbl)
      n200 = local read "LAB01-2 (A)"() -> (w301:dbl)
      n201 = local read "LAB01-2 (V)"() -> (w300:dbl)
      n202 = local read "LAB01-1 (A)"() -> (w304:dbl)
      n203 = Bundle("LAB03-1 (A)"=w297, "LAB03-1 (V)"=w296, "LAB03-1 (PF)"=w295, "LAB03-2 (A)"=w294, "LAB03-2 (V)"=w293, "LAB03-2 (PF)"=w292) -> (→"LAB03":T4)  [unwired: 1 in]
      n204 = local read "LAB05-2 (PF)"() -> (w278:dbl)
      n205 = local read "LAB05-1 (PF)"() -> (w281:dbl)
      n206 = Bundle("LAB01-1 (A)"=w304, "LAB01-1 (V)"=w303, "LAB01-1 (PF)"=w302, "LAB01-2 (A)"=w301, "LAB01-2 (V)"=w300, "LAB01-2 (PF)"=w299) -> (→"LAB01":T2)  [unwired: 1 in]
      n207 = local read "LAB05-2 (V)"() -> (w279:dbl)
      n208 = local read "LAB05-1 (A)"() -> (w283:dbl)
      n209 = local read "LAB05-1 (V)"() -> (w282:dbl)
      n210 = local read "LAB05-2 (A)"() -> (w280:dbl)
      n211 = local read "LAB04-1 (PF)"() -> (w289:dbl)
      n212 = local read "LAB04-2 (PF)"() -> (w286:dbl)
      n213 = local read "LAB04-1 (A)"() -> (w291:dbl)
      n214 = local read "LAB04-1 (V)"() -> (w290:dbl)
      n215 = local read "LAB04-2 (A)"() -> (w288:dbl)
      n216 = local read "LAB04-2 (V)"() -> (w287:dbl)
      n217 = local read "LAB02-2 (PF)"() -> (w306:dbl)
      n218 = local read "LAB02-1 (PF)"() -> (w309:dbl)
      n219 = local read "LAB02-2 (A)"() -> (w308:dbl)
      n220 = local read "LAB02-2 (V)"() -> (w307:dbl)
      n221 = local read "LAB02-1 (V)"() -> (w310:dbl)
      n222 = local read "LAB02-1 (A)"() -> (w311:dbl)
      n223 = Bundle("LAB05-1 (A)"=w283, "LAB05-1 (V)"=w282, "LAB05-1 (PF)"=w281, "LAB05-2 (A)"=w280, "LAB05-2 (V)"=w279, "LAB05-2 (PF)"=w278) -> (→"LAB05":T6)  [unwired: 1 in]
      n224 = Bundle("LAB04-1 (A)"=w291, "LAB04-1 (V)"=w290, "LAB04-1 (PF)"=w289, "LAB04-2 (A)"=w288, "LAB04-2 (V)"=w287, "LAB04-2 (PF)"=w286) -> (→"LAB04":T5)  [unwired: 1 in]
      n225 = Bundle("LAB02-1 (A)"=w311, "LAB02-1 (V)"=w310, "LAB02-1 (PF)"=w309, "LAB02-2 (A)"=w308, "LAB02-2 (V)"=w307, "LAB02-2 (PF)"=w306) -> (→"LAB02":T3)  [unwired: 1 in]
      n226 = Or(x=w272, y=w269) -> (x .or. y?=w274:bool)
      n227 = Or(x=w273, y=w268) -> (x .or. y?=w276:bool)
      n228 = Or(x=w271, y=w270) -> (x .or. y?=w275:bool)
      n229 = Build Array(w276, w274, w275) -> (→"USB Error":bool[])
    }
  }
  "array ERROR" <- w1
